vi "Get Device Property (Bool).vi"(0 "SLSC Interface in":refnum<class "SLSC Interface.lvclass">, 5 "devices":refnum<k21>="$DefaultDevices", 7 "property":refnum<k21>, 11 "error in (no error)":errorcluster) -> (4 "SLSC Interface out":refnum<class "SLSC Interface.lvclass">, 10 "property value":bool, 15 "error out":errorcluster)   [LabVIEW 2015, in "SLSC Interface.lvclass"]
uses:
  SLSC Interface.lvclass
  property type.ctl
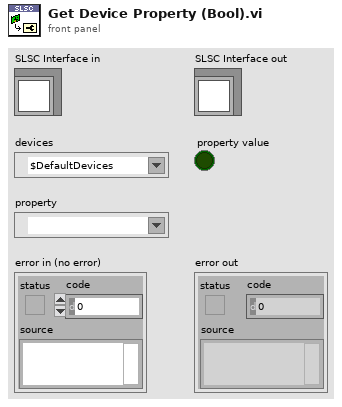
[diagram p1: front panel]
types:
  T1 = typedef "SLSC Interface.lvclass/property type.ctl" = enum16{"Bool", "DBL", "I32", "I64", "String", "U32", "U64", "1D Bool", "1D DBL", "1D I32", "1D I64", "1D String", "1D U32", "1D U64"}
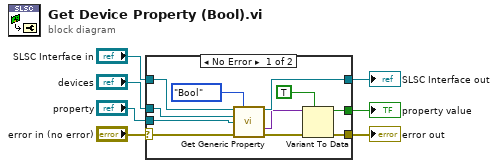
[diagram p0: block diagram]
diagram:
  n1 = case shown="No Error" "error in (no error)" {
    selector: "error in (no error)" -> [w12 w20]
    tunnel: [w11 w20] -> w6
    tunnel: [w17 w19] -> w4
    tunnel: "SLSC Interface in" -> [w18 w19]
    tunnel: [w10 _] -> w3
    tunnel: "devices" -> [w8 _]
    tunnel: "property" -> [w9 _]
    frame No Error {
      n2 = call-dynamic "Get Generic Property.vi"("SLSC Interface in"=w18, "property type"=property_type."Bool", "resources"=w8, "property"=w9, "error in (no error)"=w12) -> ("SLSC Interface out"=w17:refnum<class "SLSC Interface.lvclass">, "property value"=w15:variant, "error out"=w13:errorcluster)  [unwired: 8 in]
      n3 = Variant To Data(error in=w13, type=TRUE, Variant=w15) -> (data=w10:bool, error out=w11:errorcluster)
    }
    frame Error {
    }
  }
  "error out" <- w6
  "SLSC Interface out" <- w4
  "property value" <- w3
